vi "MSScript_SubVI_ScalarVariableAccess.vi"(4 "Init Data":cluster{"VarName":string, "VarValue":ext}[](array[cluster]), 5 "Function (Read)":enum16{"Init", "Write", "Read"}(ring)=enum."Read", 7 "VarValue":ext format="%#_13g", 9 "VarName":string) -> (0 "Value Error?":bool, 1 "OutputValue":ext, 2 "Is a variable ?":bool)   [LabVIEW 2018, in "MSScript.lvclass"]
uses:
  MSScript/MSScript.lvclass
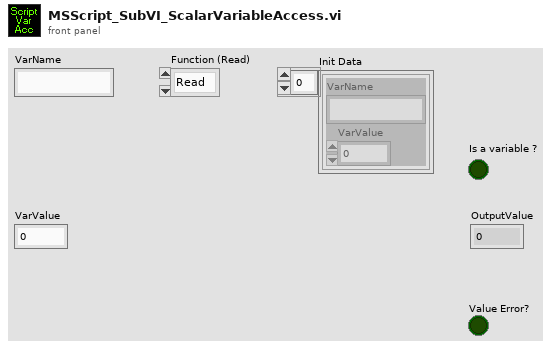
[diagram p1: front panel]
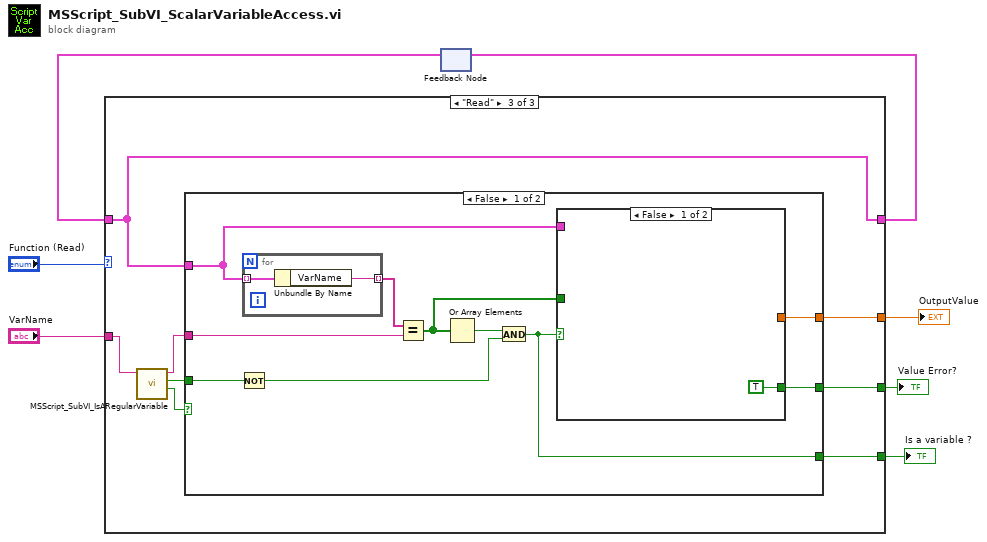
[diagram p0: block diagram]
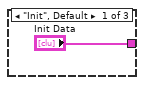
[diagram p2: hidden frame]
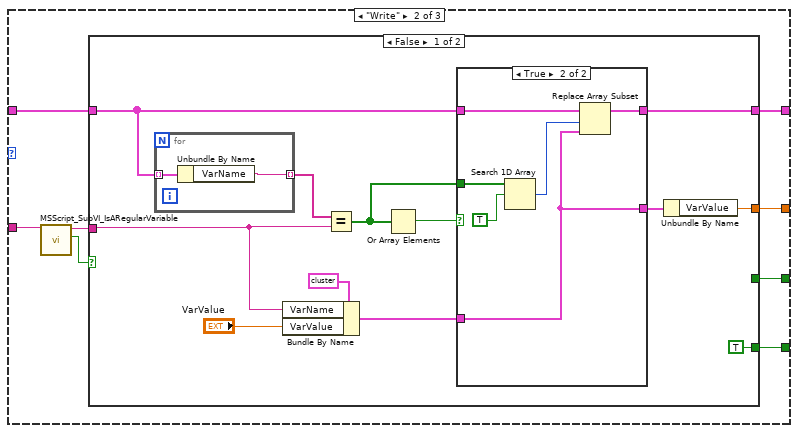
[diagram p3: hidden frame]
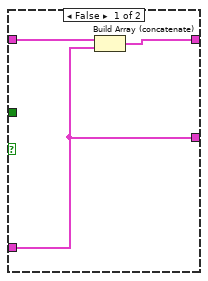
[diagram p4: hidden frame]
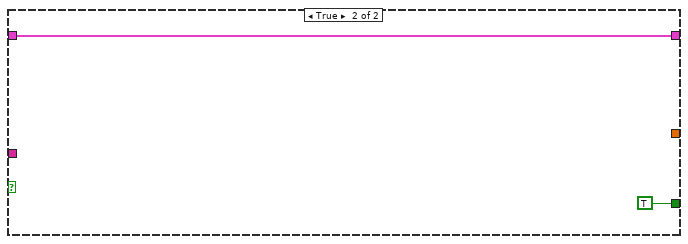
[diagram p5: hidden frame]
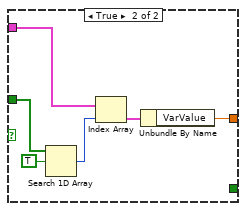
[diagram p6: hidden frame]
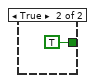
[diagram p7: hidden frame]
diagram:
  n1 = feedback #1() -> (w6:cluster{"VarName":string, "VarValue":ext}[])  [unwired: 1 in]
  n2 = case shown="\"Read\"" "Function (Read)" {
    tunnel: ["Init Data" w15 w49] -> w5
    tunnel: w6 -> [_ w16 w49]
    tunnel: "VarName" -> [_ w12 w43]
    tunnel: [_ w14 w48] -> w4
    tunnel: [_ w13 w47] -> w3
    tunnel: [_ w10 w42] -> w1
    frame "Init", Default {
    }
    frame "Write" {
      n3 = call "MSScript_SubVI_IsARegularVariable.vi"("VarString in"=w12) -> ("irregular"=w9:bool, "VarString out"=w11:string)  [unwired: 6 in, 1 out]
      n4 = case shown="False" w9 {
        tunnel: w16 -> [w26 w41]
        tunnel: [w21 w41] -> w15
        tunnel: [w20 _] -> w14
        tunnel: [_ TRUE] -> w13
        tunnel: w11 -> [w19 _]
        tunnel: [TRUE _] -> w10
        frame False {
          n5 = for {
            tunnel: w26 -> [w39] mode=indexing
            tunnel: [w38] -> w28 mode=indexing
            n6 = Unbundle By Name(w39) -> ("VarName"=w38:string)
          }
          n7 = Bundle By Name(cluster=cluster{"VarName":string, "VarValue":ext} {"VarName"="", "VarValue"=0.0} ("VariableCluster"), "VarName"=w19, "VarValue"="VarValue") -> (w25:cluster{"VarName":string, "VarValue":ext})
          n8 = Equal?(x=w28, y=w19) -> (x = y?=w27:bool[])
          n9 = Or Array Elements(Boolean array=w27) -> (logical OR=w17:bool)
          n10 = case shown="True" w17 {
            tunnel: w27 -> [_ w37]
            tunnel: w26 -> [w31 w33]
            tunnel: w25 -> [w29 w32]
            tunnel: [w30 w34] -> w21
            tunnel: [w29 w32] -> w23
            frame False {
              n11 = Build Array (concatenate)(w31, w29) -> (w30:cluster{"VarName":string, "VarValue":ext}[])
            }
            frame True {
              n12 = Search 1D Array(1D array=w37, element=TRUE) -> (index of element=w35:i32)  [unwired: 1 in]
              n13 = Replace Array Subset(array=w33, new element=w32, index=w35) -> (w34:cluster{"VarName":string, "VarValue":ext}[])
            }
          }
          n14 = Unbundle By Name(w23) -> ("VarValue"=w20:ext)
        }
        frame True {
        }
      }
    }
    frame "Read" {
      n15 = call "MSScript_SubVI_IsARegularVariable.vi"("VarString in"=w43) -> ("Variable simbol no found"=w46:bool, "irregular"=w45:bool, "VarString out"=w44:string)  [unwired: 6 in]
      n16 = case shown="False" w46 {
        tunnel: w44 -> [w57 _]
        tunnel: w49 -> [w56 _]
        tunnel: [w55 _] -> w48
        tunnel: [w54 TRUE] -> w47
        tunnel: w45 -> [w53 _]
        tunnel: [w51 _] -> w42
        frame False {
          n17 = Not(x=w53) -> (.not. x?=w52:bool)
          n18 = for {
            tunnel: [w68] -> w50 mode=indexing
            tunnel: w56 -> [w67] mode=indexing
            n19 = Unbundle By Name(w67) -> ("VarName"=w68:string)
          }
          n20 = Equal?(x=w50, y=w57) -> (x = y?=w58:bool[])
          n21 = Or Array Elements(Boolean array=w58) -> (logical OR=w59:bool)
          n22 = And(x=w59, y=w52) -> (x .and. y?=w51:bool)
          n23 = case shown="False" w51 {
            tunnel: w58 -> [_ w66]
            tunnel: w56 -> [_ w64]
            tunnel: [_ w61] -> w55
            tunnel: [TRUE _] -> w54
            frame False {
            }
            frame True {
              n24 = Search 1D Array(1D array=w66, element=TRUE) -> (index of element=w63:i32)  [unwired: 1 in]
              n25 = Index Array(array=w64, index=w63) -> (element=w62:cluster{"VarName":string, "VarValue":ext})
              n26 = Unbundle By Name(w62) -> ("VarValue"=w61:ext)
            }
          }
        }
        frame True {
        }
      }
    }
  }
  "OutputValue" <- w4
  "Value Error?" <- w3
  "Is a variable ?" <- w1
  n27 = feedback-in #1(w5) -> ()
